vi "MRC Ds Comms AccessControl Data.vi"(11 "controlFlag":u32) -> (0 "info":T1, 1 "status":cluster{"EStop":bool, "WatchdogActive":bool}, 2 "RobotMode":u8, 3 "Enabled":bool)   [LabVIEW 2026, in "MrcLib.lvlib"]
doc: "Break control flags into meaningful values"
uses:
  MrcLib.lvlib
panel:
  out "DS Connected":bool
  out "Alliance":u8
  out "TimedMatch":bool
  out "RobotWifiMode":bool
  out "SupportsOpModes":bool
  out "WatchdogActive":bool
  out "FMSConnected":bool
  out "EStop":bool
  # "breakout control flags"
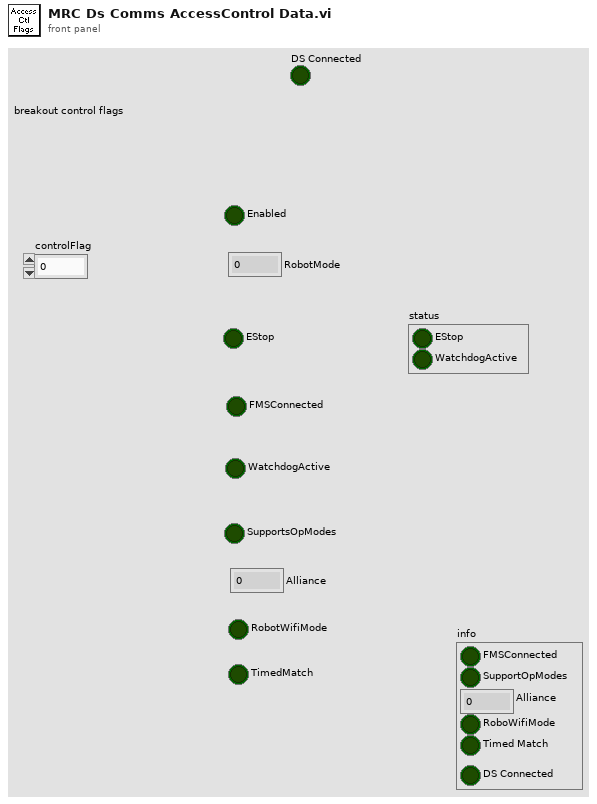
[diagram p1: front panel]
types:
  T1 = cluster{"FMSConnected":bool, "SupportOpModes":bool, "Alliance":u32, "RoboWifiMode":bool, "Timed Match":bool, "DS Connected":bool}
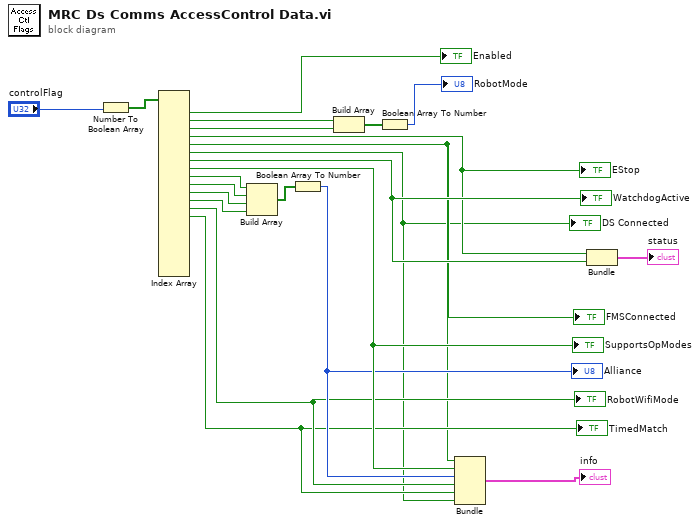
[diagram p0: block diagram]
diagram:
  n1 = Number To Boolean Array(number="controlFlag") -> (Boolean array=w21:bool[])
  n2 = Index Array(array=w21) -> (element #1=→"Enabled":bool, element #2=w5:bool, element #3=w4:bool, element #4=w3:bool, element #5=w2:bool, element #6=w1:bool, element #7=w13:bool, element #8=w12:bool, element #9=w18:bool, element #10=w17:bool, element #11=w16:bool, element #12=w15:bool, element #13=w10:bool, element #14=w9:bool)  [unwired: 21 in, 7 out]
  "EStop" <- w3
  "FMSConnected" <- w2
  "WatchdogActive" <- w13
  "SupportsOpModes" <- w12
  "RobotWifiMode" <- w10
  "TimedMatch" <- w9
  "DS Connected" <- w1
  n3 = Build Array(w18, w17, w16, w15) -> (w19:bool[])
  n4 = Boolean Array To Number(Boolean array=w19) -> (number=w11:u32)
  "Alliance" <- w11
  n5 = Build Array(w5, w4) -> (w20:bool[])
  n6 = Boolean Array To Number(Boolean array=w20) -> (number=→"RobotMode":u32)
  n7 = Bundle(w2, w12, w11, w10, w9, w1) -> (→"info":cluster{bool, bool, u32, bool, bool, bool})  [unwired: 1 in]
  n8 = Bundle(w3, w13) -> (→"status":cluster{bool, bool})  [unwired: 1 in]
